vi "Read Wheel State from Motors.vi"(8 "error in (no error)":errorcluster, 10 "wheel state in":T1, 11 "wheel in":refnum<class "NI_Robotics_Wheel.lvclass">) -> (0 "error out":errorcluster, 2 "wheel state out":T1, 3 "wheel out":refnum<class "NI_Robotics_Wheel.lvclass">)   [LabVIEW 2017, in "NI_Robotics_Wheel.lvclass"]
uses:
  <vilib>/robotics/Steering/Wheel/NI_Robotics_Wheel.lvclass
  <vilib>/robotics/Steering/Wheel/Wheel State.ctl
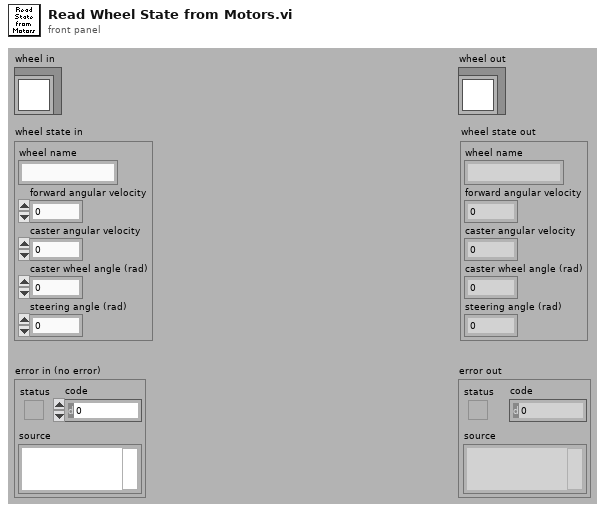
[diagram p1: front panel]
types:
  T1 = typedef "NI_Robotics_Wheel.lvclass/Wheel State.ctl" = cluster{"wheel name":string, "forward angular velocity":dbl, "caster angular velocity":dbl, "caster wheel angle (rad)":dbl, "steering angle (rad)":dbl}
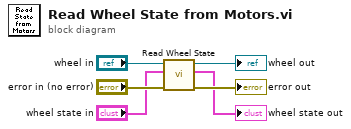
[diagram p0: block diagram]
diagram:
  n1 = call-dynamic "Read Wheel State.vi"("error in (no error)"="error in (no error)", "wheel state in"="wheel state in", "wheel in"="wheel in") -> ("error out"=→"error out":errorcluster, "wheel state out"=→"wheel state out":T1, "wheel out"=→"wheel out":refnum<class "NI_Robotics_Wheel.lvclass">)  [unwired: 6 in]
